vi "Write Anything Enhanced.vi"(7 "Format String (%#_13g)":string="%#_13g", 8 "Error In":errorcluster, 9 "Section Name (Name of \"Anything\")":string, 10 "Anything":variant, 11 "Path (dialog)":path) -> (0 "Error Out":errorcluster, 3 "Path out":path)   [LabVIEW 2020]
doc: "This VI is designed to write any data type to an INI file in human readable form. It will overwrite any data in the specified section of the INI file but leave other sections unchanged.\n\nFreeware from Moore Good Ideas, www.mooregoodideas.com. Do not remove this line."
uses:
  <vilib>/Utility/VariantDataType/VariantType.lvlib
  <vilib>/Utility/Data Type/NI_Data Type.lvlib
  Signal Synthesis VIs/3rd Generation/XControls/Stimulus Channel (G3)/Stimulus Channel (G3).xctl
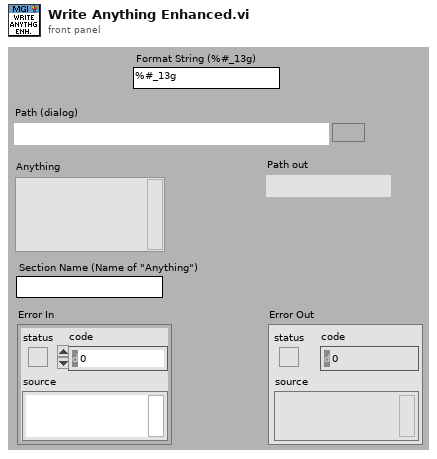
[diagram p1: front panel]
types:
  T1 = cluster{"Variant":variant, "TypeInfo":variant, "Name":string}
  T2 = typedef "NI_Data Type.lvlib/Data Type.ctl" = enum8{"Invalid Type", "Void", "I8", "I16", "I32", "I64", "U8", "U16", "U32", "U64", "Single Float", "Double Float", "Extended Float", "Single Complex", "Double Complex", "Extended Complex", "Enum U8", "Enum U16", "Enum U32", "Enum U64", "Single Float With Unit", "Double Float With Unit", "Extended Float With Unit", "Single Complex with Unit", "Double Complex with Unit", "Extended Complex with Unit", "Boolean", "String", "Path", "Picture", "Tag", "Array", "Cluster", "Variant", "LV Variant", "Waveform", "Timestamp", "Digital Waveform", "Digital Data", "ExpressData", "Refnum", "External Data", "VI", "Poly VI", "LabVIEW Class Instance", "Fixed Point", "Set Collection", "Map Collection"}
  T3 = cluster{"Variant":variant, "Variant":variant, string}
  T4 = typedef "NI_Data Type.lvlib/Type Definition Info.ctl" = cluster{"Name":string, "Timestamp":u32}
  T5 = cluster{"variant 2":variant, "variant 2":variant, string}
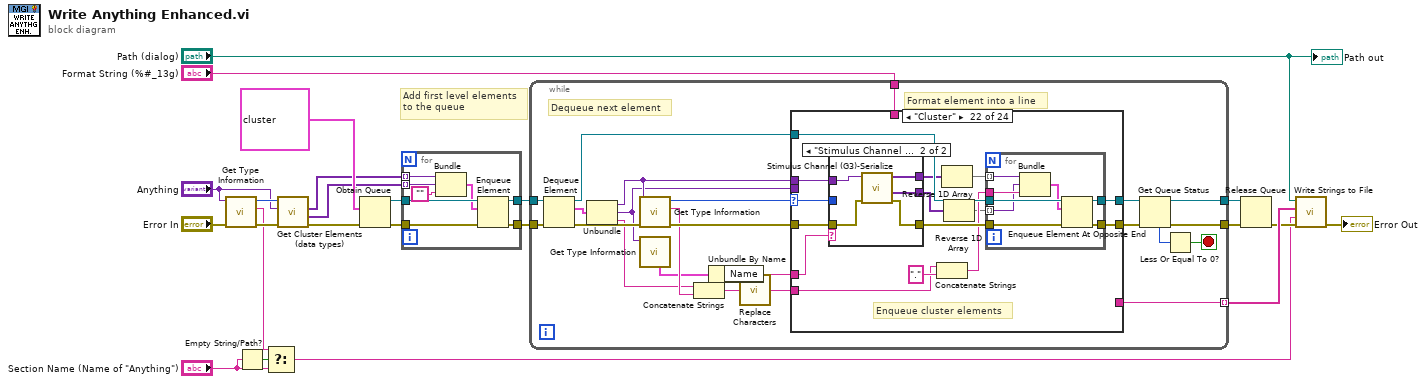
[diagram p0: block diagram]
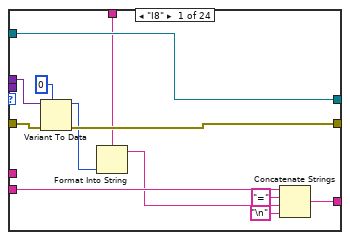
[diagram p2: hidden frame]
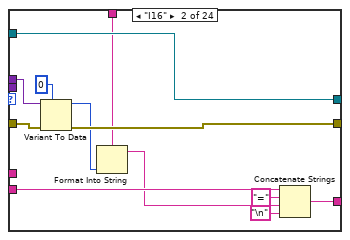
[diagram p3: hidden frame]
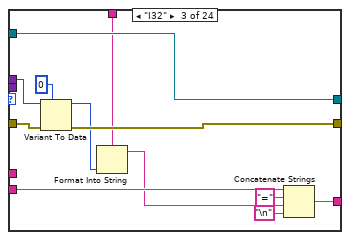
[diagram p4: hidden frame]
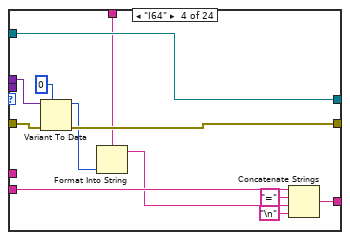
[diagram p5: hidden frame]
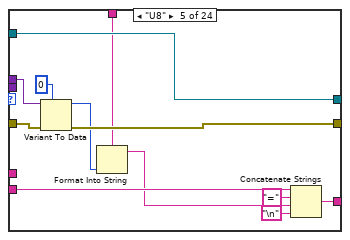
[diagram p6: hidden frame]
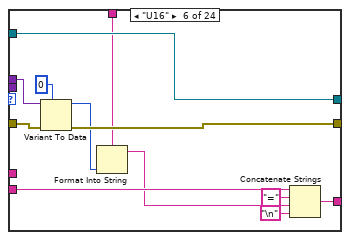
[diagram p7: hidden frame]
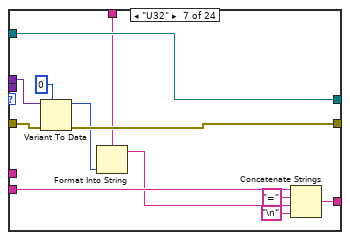
[diagram p8: hidden frame]
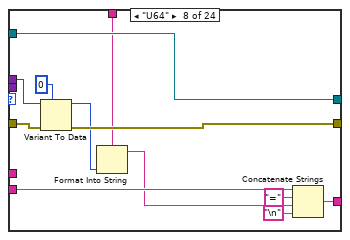
[diagram p9: hidden frame]
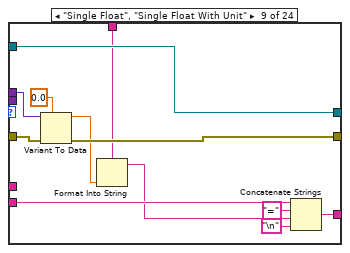
[diagram p10: hidden frame]
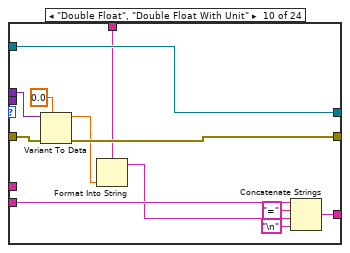
[diagram p11: hidden frame]
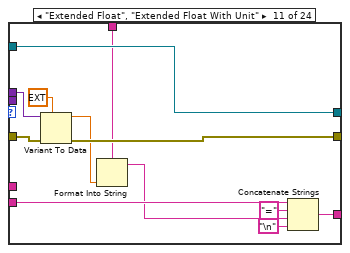
[diagram p12: hidden frame]
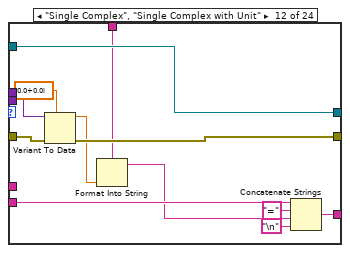
[diagram p13: hidden frame]
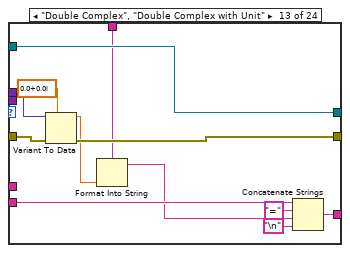
[diagram p14: hidden frame]
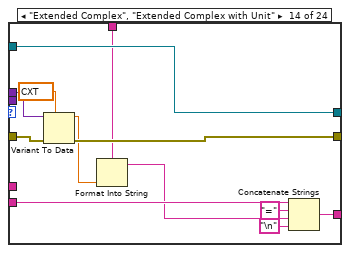
[diagram p15: hidden frame]
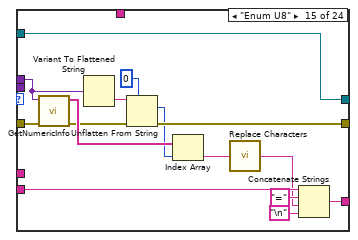
[diagram p16: hidden frame]
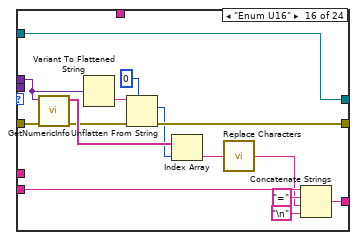
[diagram p17: hidden frame]
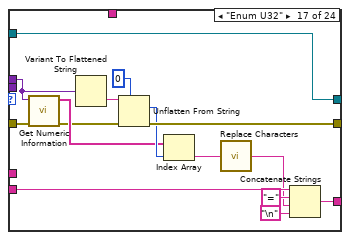
[diagram p18: hidden frame]
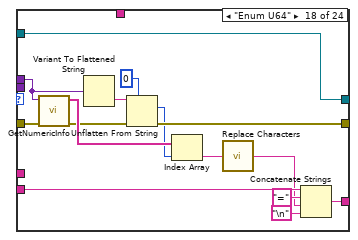
[diagram p19: hidden frame]
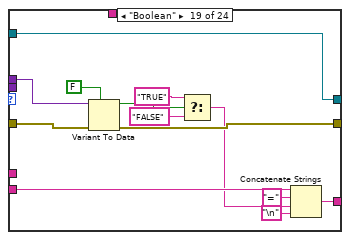
[diagram p20: hidden frame]
diagram:
  # "Add first level elements\nto the queue"
  n1 = call <vilib>:"Get Type Information.vi"("error in (no error)"="Error In", "variant"="Anything") -> ("error out"=w5:errorcluster, "name"=w4:string, "type"=w6:T2)  [unwired: 5 in, 2 out]
  n2 = Empty String/Path?(string/path="Section Name (Name of \"Anything\")") -> (empty?=w11:bool)
  n3 = Select(t=w4, s=w11, f="Section Name (Name of \"Anything\")") -> (s? t:f=w9:string)
  n4 = call "Get Cluster Elements (data types).vi"("Error In"=w5, "Cluster"="Anything", "Type Enum (Cluster)"=w6) -> ("Error Out"=w15:errorcluster, "Types Out"=w1:variant[], "Cluster Elements"=w2:variant[])  [unwired: 6 in]
  n5 = Obtain Queue(element data type=T1 {"Variant"=variant, "TypeInfo"=variant, "Name"=""}, error in (no error)=w15) -> (queue out=w22:refnum<queue>, error out=w21:errorcluster)  [unwired: 3 in, 1 out]
  n6 = for {
    tunnel: w22 -> [w31]
    tunnel: w21 -> [w30]
    tunnel: [w29] -> w20
    tunnel: [w28] -> w19
    tunnel: w2 -> [w26] mode=indexing
    tunnel: w1 -> [w24] mode=indexing
    n7 = Bundle("Variant"=w26, "Variant"=w24, "") -> (w27:T3)  [unwired: 1 in]
    n8 = Enqueue Element(queue=w31, element=w27, error in (no error)=w30) -> (queue out=w28:refnum<queue>, error out=w29:errorcluster)  [unwired: 1 in, 1 out]
  }
  n9 = while {
    tunnel: w20 -> [w54]
    tunnel: [w52] -> w18
    tunnel: [w44] -> w23 mode=indexing
    tunnel: w19 -> [w53]
    tunnel: [w49] -> w17
    tunnel: "Format String (%#_13g)" -> [w41]
    stop <- w50 stop-if-true
    # "Format element into a line"
    # "Dequeue next element"
    n10 = Dequeue Element(queue=w53, error in (no error)=w54) -> (queue out=w47:refnum<queue>, element=w45:T1, error out=w40:errorcluster)  [unwired: 1 in, 1 out]
    n11 = Unbundle(w45) -> ("Variant"=w34:variant, "TypeInfo"=w32:variant, "Name"=w35:string)
    n12 = call <vilib>:"Get Type Information.vi"("error in (no error)"=w40, "variant"=w34) -> ("error out"=w39:errorcluster, "name"=w38:string, "type"=w37:T2)  [unwired: 5 in, 2 out]
    n13 = call <vilib>:"Get Type Information.vi"("variant"=w32) -> ("type definition info"=w33:T4)  [unwired: 6 in, 4 out]
    n14 = Concatenate Strings(w35, w38) -> (w43:string)
    n15 = Unbundle By Name(w33) -> ("Name"=w36:string)
    n16 = call "Replace Characters.vi"("String In"=w43) -> ("String Out"=w42:string)  [unwired: 1 in]
    n17 = case shown="\"Cluster\"" w37 {
      selector: w37 -> [_ _ _ _ _ _ _ _ _ _ _ _ _ _ _ _ _ _ _ _ _ w327 _ _]
      tunnel: [w66 w78 w90 w102 w114 w126 w138 w150 w162 w174 w186 w198 w210 w222 w237 w252 w267 w282 w295 w306 w318 w331 w354 w377] -> w48
      tunnel: w47 -> [w66 w78 w90 w102 w114 w126 w138 w150 w162 w174 w186 w198 w210 w222 w237 w252 w267 w282 w295 w306 w318 w332 w355 w377]
      tunnel: [w62 w74 w86 w98 w110 w122 w134 w146 w158 w170 w182 w194 w206 w218 w231 w246 w265 w276 w294 w305 w317 w333 w362 w376] -> w46
      tunnel: w39 -> [w65 w77 w89 w101 w113 w125 w137 w149 w161 w173 w185 w197 w209 w221 w236 w251 w256 w281 w291 w302 w314 w329 w363 w376]
      tunnel: w42 -> [w59 w70 w82 w94 w106 w118 w130 w142 w154 w166 w178 w189 w201 w213 w225 w240 w259 w270 w284 w298 w309 w323 w358 w366]
      tunnel: w34 -> [w64 w76 w88 w100 w112 w124 w136 w148 w160 w172 w184 w196 w208 w220 w234 w249 w255 w279 w292 w303 w315 w326 w364 w375]
      tunnel: [w58 w71 w83 w95 w107 w119 w131 w143 w155 w167 w179 w190 w202 w214 w226 w241 w260 w271 w285 w299 w310 _ w359 w367] -> w44
      tunnel: w41 -> [w55 w67 w79 w93 w103 w115 w127 w139 w151 w164 w175 w187 w199 w211 _ _ _ _ _ _ _ _ w356 _]
      tunnel: w36 -> [_ _ _ _ _ _ _ _ _ _ _ _ _ _ _ _ _ _ _ _ _ w321 _ _]
      tunnel: w32 -> [_ _ _ _ _ _ _ _ _ _ _ _ _ _ _ _ _ _ _ _ _ _ w353 _]
      frame "I8" {
        n18 = Variant To Data(error in=w65, type=i8 0, Variant=w64) -> (data=w57:i8, error out=w62:errorcluster)
        n19 = Format Into String(format string=w55, w57) -> (resulting string=w56:string)  [unwired: 2 in, 1 out]
        n20 = Concatenate Strings(w59, "=" ("string"), w56, "\n") -> (w58:string)
      }
      frame "I16" {
        n21 = Variant To Data(error in=w77, type=i16 0, Variant=w76) -> (data=w68:i16, error out=w74:errorcluster)
        n22 = Format Into String(format string=w67, w68) -> (resulting string=w69:string)  [unwired: 2 in, 1 out]
        n23 = Concatenate Strings(w70, "=" ("string"), w69, "\n") -> (w71:string)
      }
      frame "I32" {
        n24 = Variant To Data(error in=w89, type=0, Variant=w88) -> (data=w81:i32, error out=w86:errorcluster)
        n25 = Format Into String(format string=w79, w81) -> (resulting string=w80:string)  [unwired: 2 in, 1 out]
        n26 = Concatenate Strings(w82, "=" ("string"), w80, "\n") -> (w83:string)
      }
      frame "I64" {
        n27 = Variant To Data(error in=w101, type=i64 0, Variant=w100) -> (data=w92:i64, error out=w98:errorcluster)
        n28 = Format Into String(format string=w93, w92) -> (resulting string=w91:string)  [unwired: 2 in, 1 out]
        n29 = Concatenate Strings(w94, "=" ("string"), w91, "\n") -> (w95:string)
      }
      frame "U8" {
        n30 = Variant To Data(error in=w113, type=u8 0, Variant=w112) -> (data=w105:u8, error out=w110:errorcluster)
        n31 = Format Into String(format string=w103, w105) -> (resulting string=w104:string)  [unwired: 2 in, 1 out]
        n32 = Concatenate Strings(w106, "=" ("string"), w104, "\n") -> (w107:string)
      }
      frame "U16" {
        n33 = Variant To Data(error in=w125, type=u16 0, Variant=w124) -> (data=w117:u16, error out=w122:errorcluster)
        n34 = Format Into String(format string=w115, w117) -> (resulting string=w116:string)  [unwired: 2 in, 1 out]
        n35 = Concatenate Strings(w118, "=" ("string"), w116, "\n") -> (w119:string)
      }
      frame "U32" {
        n36 = Variant To Data(error in=w137, type=u32 0, Variant=w136) -> (data=w129:u32, error out=w134:errorcluster)
        n37 = Format Into String(format string=w127, w129) -> (resulting string=w128:string)  [unwired: 2 in, 1 out]
        n38 = Concatenate Strings(w130, "=" ("string"), w128, "\n") -> (w131:string)
      }
      frame "U64" {
        n39 = Variant To Data(error in=w149, type=u64 0, Variant=w148) -> (data=w141:u64, error out=w146:errorcluster)
        n40 = Format Into String(format string=w139, w141) -> (resulting string=w140:string)  [unwired: 2 in, 1 out]
        n41 = Concatenate Strings(w142, "=" ("string"), w140, "\n") -> (w143:string)
      }
      frame "Single Float", "Single Float With Unit" {
        n42 = Variant To Data(error in=w161, type=sgl 0.0, Variant=w160) -> (data=w153:sgl, error out=w158:errorcluster)
        n43 = Format Into String(format string=w151, w153) -> (resulting string=w152:string)  [unwired: 2 in, 1 out]
        n44 = Concatenate Strings(w154, "=" ("string"), w152, "\n") -> (w155:string)
      }
      frame "Double Float", "Double Float With Unit" {
        n45 = Variant To Data(error in=w173, type=0.0, Variant=w172) -> (data=w165:dbl, error out=w170:errorcluster)
        n46 = Format Into String(format string=w164, w165) -> (resulting string=w163:string)  [unwired: 2 in, 1 out]
        n47 = Concatenate Strings(w166, "=" ("string"), w163, "\n") -> (w167:string)
      }
      frame "Extended Float", "Extended Float With Unit" {
        n48 = Variant To Data(error in=w185, type=ext 0.0, Variant=w184) -> (data=w177:ext, error out=w182:errorcluster)
        n49 = Format Into String(format string=w175, w177) -> (resulting string=w176:string)  [unwired: 2 in, 1 out]
        n50 = Concatenate Strings(w178, "=" ("string"), w176, "\n") -> (w179:string)
      }
      frame "Single Complex", "Single Complex with Unit" {
        n51 = Variant To Data(error in=w197, type=csg 0.0+0.0i, Variant=w196) -> (data=w193:csg, error out=w194:errorcluster)
        n52 = Format Into String(format string=w187, w193) -> (resulting string=w188:string)  [unwired: 2 in, 1 out]
        n53 = Concatenate Strings(w189, "=" ("string"), w188, "\n") -> (w190:string)
      }
      frame "Double Complex", "Double Complex with Unit" {
        n54 = Variant To Data(error in=w209, type=cdb 0.0+0.0i, Variant=w208) -> (data=w205:cdb, error out=w206:errorcluster)
        n55 = Format Into String(format string=w199, w205) -> (resulting string=w200:string)  [unwired: 2 in, 1 out]
        n56 = Concatenate Strings(w201, "=" ("string"), w200, "\n") -> (w202:string)
      }
      frame "Extended Complex", "Extended Complex with Unit" {
        n57 = Variant To Data(error in=w221, type=cxt 0.0+0.0i, Variant=w220) -> (data=w217:cxt, error out=w218:errorcluster)
        n58 = Format Into String(format string=w211, w217) -> (resulting string=w212:string)  [unwired: 2 in, 1 out]
        n59 = Concatenate Strings(w213, "=" ("string"), w212, "\n") -> (w214:string)
      }
      frame "Enum U8" {
        n60 = call <vilib>:"GetNumericInfo.vi"("error in (no error)"=w236, "Variant"=w234) -> ("error out"=w232:errorcluster, "EnumNames"=w235:string[])  [unwired: 6 in, 2 out]
        n61 = Variant To Flattened String(Variant=w234) -> (data string=w233:string)  [unwired: 1 out]
        n62 = Unflatten From String(type=u8 0, binary string=w233, error in (no error)=w232) -> (value=w230:u8, error out=w231:errorcluster)  [unwired: 2 in, 1 out]
        n63 = Index Array(array=w235, index=w230) -> (element=w224:string)
        n64 = call "Replace Characters.vi"("String In"=w224) -> ("String Out"=w223:string)  [unwired: 1 in]
        n65 = Concatenate Strings(w225, "=" ("string"), w223, "\n") -> (w226:string)
      }
      frame "Enum U16" {
        n66 = call <vilib>:"GetNumericInfo.vi"("error in (no error)"=w251, "Variant"=w249) -> ("error out"=w247:errorcluster, "EnumNames"=w250:string[])  [unwired: 6 in, 2 out]
        n67 = Variant To Flattened String(Variant=w249) -> (data string=w248:string)  [unwired: 1 out]
        n68 = Unflatten From String(type=u16 0, binary string=w248, error in (no error)=w247) -> (value=w245:u16, error out=w246:errorcluster)  [unwired: 2 in, 1 out]
        n69 = Index Array(array=w250, index=w245) -> (element=w239:string)
        n70 = call "Replace Characters.vi"("String In"=w239) -> ("String Out"=w238:string)  [unwired: 1 in]
        n71 = Concatenate Strings(w240, "=" ("string"), w238, "\n") -> (w241:string)
      }
      frame "Enum U32" {
        n72 = call <vilib>:"Get Numeric Information.vi"("error in (no error)"=w256, "variant"=w255) -> ("error out"=w253:errorcluster, "enum names"=w254:string[])  [unwired: 6 in, 2 out]
        n73 = Variant To Flattened String(Variant=w255) -> (data string=w266:string)  [unwired: 1 out]
        n74 = Unflatten From String(type=u32 0, binary string=w266, error in (no error)=w253) -> (value=w264:u32, error out=w265:errorcluster)  [unwired: 2 in, 1 out]
        n75 = Index Array(array=w254, index=w264) -> (element=w258:string)
        n76 = call "Replace Characters.vi"("String In"=w258) -> ("String Out"=w257:string)  [unwired: 1 in]
        n77 = Concatenate Strings(w259, "=" ("string"), w257, "\n") -> (w260:string)
      }
      frame "Enum U64" {
        n78 = call <vilib>:"GetNumericInfo.vi"("error in (no error)"=w281, "Variant"=w279) -> ("error out"=w277:errorcluster, "EnumNames"=w280:string[])  [unwired: 6 in, 2 out]
        n79 = Variant To Flattened String(Variant=w279) -> (data string=w278:string)  [unwired: 1 out]
        n80 = Unflatten From String(type=u64 0, binary string=w278, error in (no error)=w277) -> (value=w275:u64, error out=w276:errorcluster)  [unwired: 2 in, 1 out]
        n81 = Index Array(array=w280, index=w275) -> (element=w269:string)
        n82 = call "Replace Characters.vi"("String In"=w269) -> ("String Out"=w268:string)  [unwired: 1 in]
        n83 = Concatenate Strings(w270, "=" ("string"), w268, "\n") -> (w271:string)
      }
      frame "Boolean" {
        n84 = Variant To Data(error in=w291, type=FALSE, Variant=w292) -> (data=w290:bool, error out=w294:errorcluster)
        n85 = Select(t="TRUE", s=w290, f="FALSE") -> (s? t:f=w283:string)
        n86 = Concatenate Strings(w284, "=" ("string"), w283, "\n") -> (w285:string)
      }
      frame "String" {
        n87 = Variant To Data(error in=w302, type="", Variant=w303) -> (data=w297:string, error out=w305:errorcluster)
        n88 = call "Replace Characters.vi"("String In"=w297) -> ("String Out"=w296:string)  [unwired: 1 in]
        n89 = Concatenate Strings(w298, "=" ("string"), w296, "\n") -> (w299:string)
      }
      frame "Path" {
        n90 = Variant To Data(error in=w314, type=path "", Variant=w315) -> (data=w313:path, error out=w317:errorcluster)
        n91 = Path To String(path=w313) -> (string=w308:string)
        n92 = call "Replace Characters.vi"("String In"=w308) -> ("String Out"=w307:string)  [unwired: 1 in]
        n93 = Concatenate Strings(w309, "=" ("string"), w307, "\n") -> (w310:string)
      }
      frame "Cluster" {
        # "Enqueue cluster elements"
        n94 = case shown="\"Stimulus Channel (G3).xctl:Full Stimulus Channel Data.ctl\"" w321 {
          tunnel: w329 -> [w339 w341]
          tunnel: [w338 w340] -> w328
          tunnel: w327 -> [w337 _]
          tunnel: w326 -> [w336 w344]
          tunnel: [w335 w343] -> w325
          tunnel: [w334 w342] -> w320
          frame "Default", Default {
            n95 = call "Get Cluster Elements (data types).vi"("Error In"=w339, "Cluster"=w336, "Type Enum (Cluster)"=w337) -> ("Error Out"=w338:errorcluster, "Types Out"=w334:variant[], "Cluster Elements"=w335:variant[])  [unwired: 6 in]
          }
          frame "Stimulus Channel (G3).xctl:Full Stimulus Channel Data.ctl" {
            n96 = call "Stimulus Channel (G3)-Serialize.vi"("error in"=w341, "variant"=w344) -> ("error out"=w340:errorcluster, "Cluster Data Types"=w342:variant[], "Cluster Variants"=w343:variant[])  [unwired: 7 in]
          }
        }
        n97 = Concatenate Strings(w323, "." ("string")) -> (w322:string)
        n98 = Reverse 1D Array(array=w325) -> (reversed array=w330:variant[])
        n99 = Reverse 1D Array(array=w320) -> (reversed array=w319:variant[])
        n100 = for {
          tunnel: w332 -> [w352]
          tunnel: w328 -> [w351]
          tunnel: [w350] -> w333
          tunnel: [w349] -> w331
          tunnel: w330 -> [w348] mode=indexing
          tunnel: w322 -> [w347]
          tunnel: w319 -> [w345] mode=indexing
          n101 = Bundle("variant 2"=w348, "variant 2"=w345, w347) -> (w346:T5)  [unwired: 1 in]
          n102 = Enqueue Element At Opposite End(queue=w352, element=w346, error in (no error)=w351) -> (queue out=w349:refnum<queue>, error out=w350:errorcluster)  [unwired: 1 in, 1 out]
        }
      }
      frame "Array" {
        n103 = call "Process Array Elements (data types).vi"("Queue In"=w355, "Format String (%#0.15f)"=w356, "Array Variant"=w364, "Data type"=w353, "Name In"=w358, "Error In"=w363) -> ("Queue Out"=w354:refnum<queue>, "Data Out"=w357:string, "Error Out"=w362:errorcluster)  [unwired: 7 in]
        n104 = Concatenate Strings(w358, "=" ("string"), w357, "\n") -> (w359:string)
      }
      frame Default {
        n105 = Variant To Flattened String(Variant=w375) -> (data string=w370:string)  [unwired: 1 out]
        n106 = String To Byte Array(string=w370) -> (unsigned byte array=w374:u8[])
        n107 = Number To Hexadecimal String(1:i16 2 ("width (-)"), 2:w374) -> (0:w373:string[])
        n108 = Concatenate Strings("0x", w373) -> (w365:string)
        n109 = Concatenate Strings(w366, "=" ("string"), w365, "\n") -> (w367:string)
      }
    }
    n110 = Get Queue Status(queue=w48, error in (no error)=w46) -> (queue out=w49:refnum<queue>, error out=w52:errorcluster, # elements in queue=w51:i32)  [unwired: 1 in, 5 out]
    n111 = Less Or Equal To 0?(x=w51) -> (x <= 0?=w50:bool)
  }
  n112 = Release Queue(queue=w17, error in (no error)=w18) -> (error out=w13:errorcluster)  [unwired: 1 in, 2 out]
  n113 = call "Write Strings to File.vi"("Error In"=w13, "Section Name"=w9, "Array of Strings"=w23, "Path"="Path (dialog)") -> ("Error Out"=→"Error Out":errorcluster)  [unwired: 7 in]
  "Path out" <- "Path (dialog)"
